vi "circularMovimentOrientationTest.vi"(8 "error in (no error)":errorcluster, 10 "robotPostion":dbl[](array[numeric]), 11 "Game in":refnum<class "Game.lvclass">) -> (0 "error out":errorcluster, 2 "dest_orientation":dbl, 3 "Game out":refnum<class "Game.lvclass">)   [LabVIEW 2020, in "Game.lvclass"]
uses:
  Game.lvclass
  <vilib>/Analysis/coordinate.llb/2D Cartesian Coordinate Rotation (Scalar).vi
  <vilib>/Analysis/NI_AALPro.lvlib
panel:
  out "debug orient":dbl
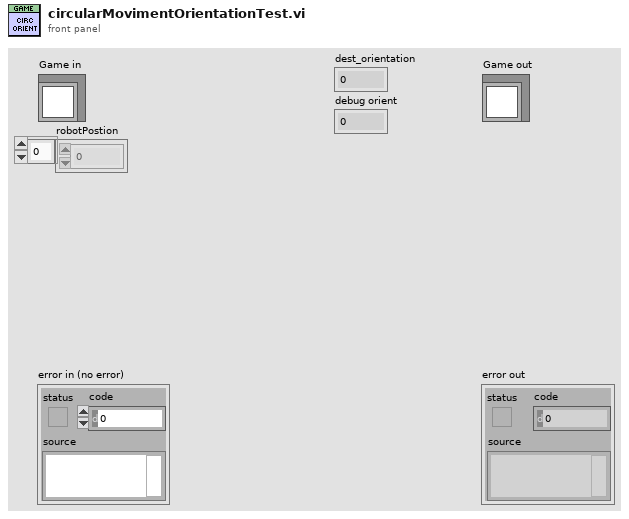
[diagram p1: front panel]
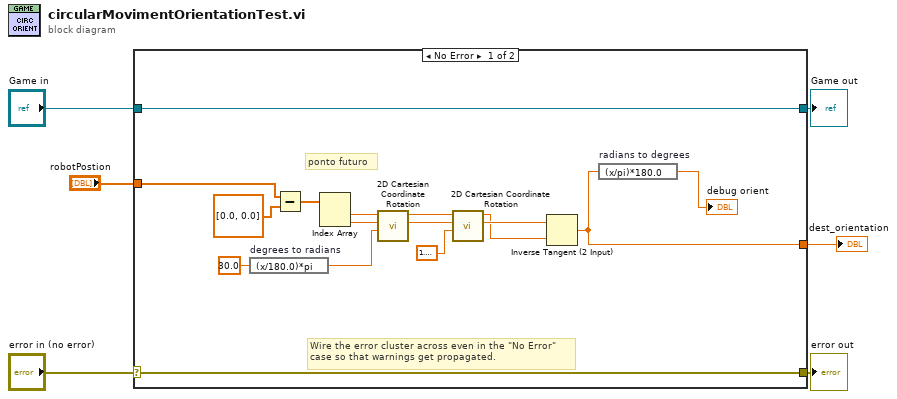
[diagram p0: block diagram]
diagram:
  n1 = case shown="No Error" "error in (no error)" {
    selector: "error in (no error)" -> [w21 w24]
    tunnel: [w21 w24] -> w5
    tunnel: [w22 w23] -> w3
    tunnel: "Game in" -> [w22 w23]
    tunnel: "robotPostion" -> [w17 _]
    tunnel: [w15 _] -> w1
    frame No Error {
      # "ponto futuro"
      # "Wire the error cluster across even in the \"No Error\"\ncase so that warnings get propagated."
      n2 = expression code="(x/180.0)*pi" "degrees to radians"(30.0) -> (w13:dbl)
      n3 = Subtract(x=w17, y=dbl[] [0.0, 0.0]) -> (x-y=w16:dbl[])
      n4 = Index Array(array=w16) -> (element #1=w19:dbl, element #2=w20:dbl)  [unwired: 2 in]
      n5 = call-poly <vilib>:"2D Cartesian Coordinate Rotation.vi"("theta"=w13, "y"=w20, "x"=w19) -> ("y out"=w10:dbl, "x out"=w11:dbl)  [unwired: 6 in, 1 out]
      n6 = call-poly <vilib>:"2D Cartesian Coordinate Rotation.vi"("theta"=1.5707963267948966, "y"=w10, "x"=w11) -> ("y out"=w8:dbl, "x out"=w7:dbl)  [unwired: 6 in, 1 out]
      n7 = Inverse Tangent (2 Input)(1:w7, 2:w8) -> (0:w15:dbl)
      n8 = expression code="(x/pi)*180.0" "radians to degrees"(w15) -> (→"debug orient":dbl)
    }
    frame Error {
    }
  }
  "error out" <- w5
  "Game out" <- w3
  "dest_orientation" <- w1
